vi "Write HVAC Control.vi"(8 "error in":errorcluster, 10 "HVAC_Control":T1, 11 "HVAC in":refnum<class "HVAC.lvclass">) -> (0 "error out":errorcluster, 3 "HVAC out":refnum<class "HVAC.lvclass">)   [LabVIEW 2018, in "HVAC Actor.lvlib" / "HVAC.lvclass"]
uses:
  HVAC.lvclass
  C:/Users/Administrator/Desktop/2018LabVIEW EMS/IED Actors/Device DDS Communications Framework/Device DDS Communications/Device DDS Communications.lvclass
  <vilib>/ORNL/CSEISMIC DDS/CSEISMIC DDS Base/Data Types/HVAC_Control.ctl
  <vilib>/ORNL/CSEISMIC DDS/CSEISMIC DDS Base/Data Types/Controls/DeviceID.ctl
  <vilib>/ORNL/CSEISMIC DDS/CSEISMIC DDS Base/Data Types/Controls/ControlMode.ctl
  Device DDS Communications Framework/Device DDS Communications/Device DDS Communications.lvclass/Device DDS Communications.ctl
  <vilib>/ORNL/CSEISMIC DDS/CSEISMIC DDS Base/CSEISMIC DDS.lvclass/CSEISMIC DDS.ctl
  <vilib>/ORNL/CSEISMIC DDS/CSEISMIC DDS Base/Accessors/Read DDS Reference.vi
  <vilib>/ORNL/CSEISMIC DDS/DDS Writer/DDS Writer.lvclass
  C:/Program Files (x86)/National Instruments/LabVIEW 2018/vi.lib/ORNL/CSEISMIC DDS/CSEISMIC DDS Base/CSEISMIC DDS.lvclass
  <vilib>/ORNL/CSEISMIC DDS/CSEISMIC DDS Base/Error Handler.vi
  Device DDS Communications Framework/Device DDS Communications/Device DDS Communications.lvclass
  <vilib>/ORNL/CSEISMIC DDS/CSEISMIC DDS Base/CSEISMIC DDS.lvclass
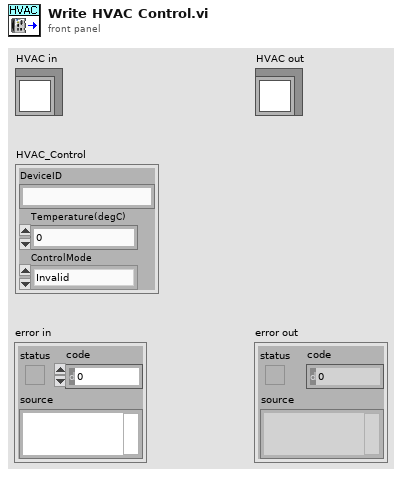
[diagram p1: front panel]
types:
  T1 = typedef "CSEISMIC DDS.lvlib/CSEISMIC DDS.lvclass/HVAC_Control.ctl" = cluster{"DeviceID":T2, "Temperature(degC)":dbl, "ControlMode":T3}
  T2 = typedef "CSEISMIC DDS.lvlib/CSEISMIC DDS.lvclass/DeviceID.ctl" = string
  T3 = typedef "CSEISMIC DDS.lvlib/CSEISMIC DDS.lvclass/ControlMode.ctl" = enum32{"Invalid", "Cooling", "Heating"}
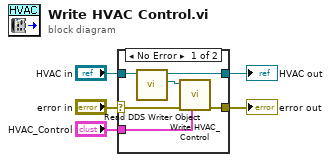
[diagram p0: block diagram]
diagram:
  n1 = case shown="No Error" "error in" {
    selector: "error in" -> [w8 w13]
    tunnel: [w6 w13] -> w4
    tunnel: [w10 w12] -> w2
    tunnel: "HVAC in" -> [w11 w12]
    tunnel: "HVAC_Control" -> [w7 _]
    frame No Error {
      n2 = call "Read DDS Writer Object.vi"("Device DDS Communications in"=w11) -> ("DDS Writer Object"=w9:refnum<class "DDS Writer.lvclass">, "Device DDS Communications out"=w10:refnum<class "HVAC.lvclass">)  [unwired: 9 in]
      n3 = call <vilib>:"Write HVAC_Control.vi"("HVAC_Control"=w7, "error in"=w8, "DDS Writer in"=w9) -> ("error out"=w6:errorcluster)  [unwired: 7 in, 1 out]
    }
    frame Error {
    }
  }
  "error out" <- w4
  "HVAC out" <- w2
